vi "Add Package to SystemLink Feed.vi"() -> ()   [LabVIEW 2017, in "SystemLink_Repo_API.lvlib"]
doc: "This example shows how to upload and add a package to a SystemLink feed."
uses:
  SystemLink_Repo_API.lvlib
  Open SystemLink Connection (API Key).vi
  Open SystemLink Connection (Basic).vi
panel:
  in  "Login Options":enum32{"Username and Password", "API Key"}(tab)
  in  "Username":string
  in  "Password":string
  in  "API Key":string
  out "Packages in the specified feed":string[][](table)
  in  "SystemLink Feed Name":string
  in  "Package Filepath":path
  in  "SystemLink server base URL":string="https://"
  # "SystemLink Server"
  # "Package to Add to SystemLink Feed"
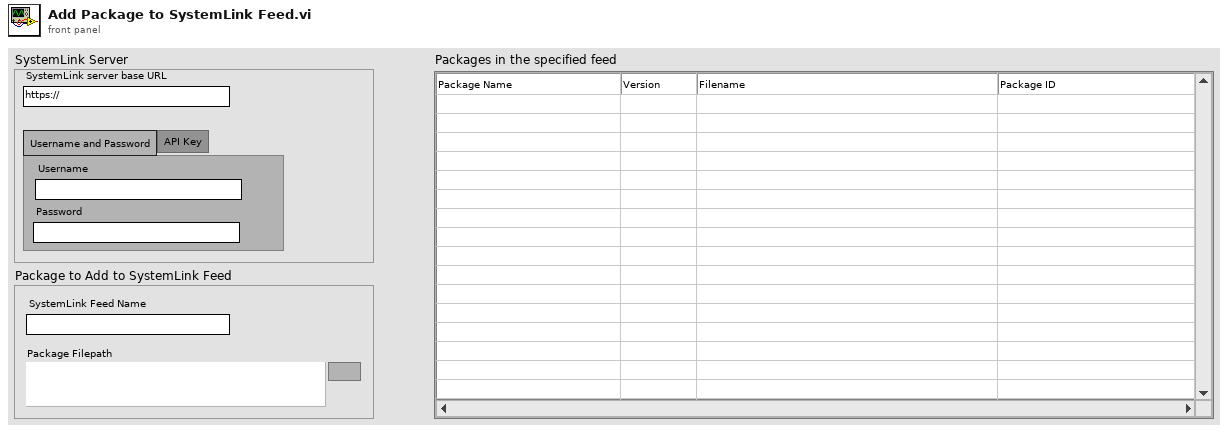
[diagram p1: front panel]
types:
  T1 = typedef "SystemLink_Repo_API.lvlib/systemlink repo.ctl" = cluster{"client handle out":T2, "SystemLink server base URL":string}
  T2 = typedef "LabVIEWHTTPClient.lvlib/ClientHandle.ctl" = refnum<k1>
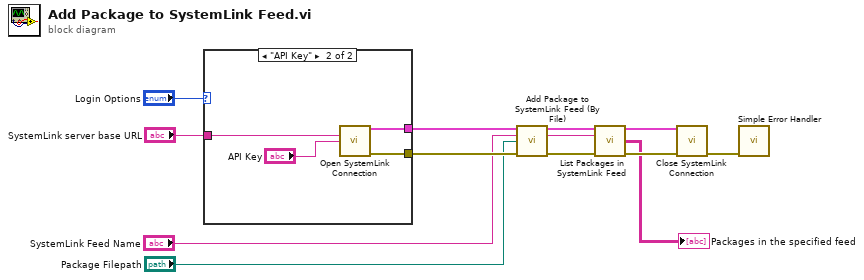
[diagram p0: block diagram]
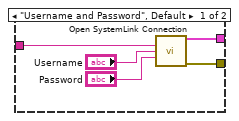
[diagram p2: hidden frame]
diagram:
  n1 = case shown="\"API Key\"" "Login Options" {
    tunnel: [w18 w22] -> w13
    tunnel: [w17 w21] -> w12
    tunnel: "SystemLink server base URL" -> [w14 w20]
    frame "Username and Password", Default {
      n2 = call-poly "Open SystemLink Connection.vi"("SystemLink server base URL"=w14, "username"="Username", "password"="Password") -> ("SystemLink repo out"=w18:T1, "error out"=w17:errorcluster)  [unwired: 11 in]
    }
    frame "API Key" {
      n3 = call-poly "Open SystemLink Connection.vi"("SystemLink server base URL"=w20, "API Key"="API Key") -> ("SystemLink repo out"=w22:T1, "error out"=w21:errorcluster)  [unwired: 12 in]
    }
  }
  n4 = call "Add Package to SystemLink Feed (By File).vi"("SystemLink repo in"=w13, "feed name in"="SystemLink Feed Name", "package filepath"="Package Filepath", "error in (no error)"=w12) -> ("SystemLink repo out"=w7:T1, "feed name out"=w3:string, "error out"=w5:errorcluster)  [unwired: 8 in, 1 out]
  n5 = call "List Packages in SystemLink Feed.vi"("SystemLink repo in"=w7, "feed name in"=w3, "error in (no error)"=w5) -> ("SystemLink repo out"=w6:T1, "packages"=→"Packages in the specified feed":string[][], "error out"=w4:errorcluster)  [unwired: 9 in, 1 out]
  n6 = call "Close SystemLink Connection.vi"("SystemLink repo in"=w6, "error in (no error)"=w4) -> ("error out"=w10:errorcluster)  [unwired: 13 in]
  n7 = call <vilib>:"Simple Error Handler.vi"("error in (no error)"=w10) -> ()  [unwired: 4 in, 5 out]
